vi "UpdateDAQLinescanImage.vi"(2 "Image Settings":refnum<vi>, 3 "buffer (output)":u32[](array[numeric]), 4 "count (read)":u32, 5 "operation":enum16{"initialize", "update", "read"}(ring)) -> (0 "LinescanSampling":T1 {"MacrotimeCycle" format="%.2f"; "OverflowConstant" format="%.2f"; "BinningMicroS" format="%.2f"}, 1 "end of line":bool)   [LabVIEW 2009]
uses:
  ImageSettings.ctt
  ScannedImage.ctl
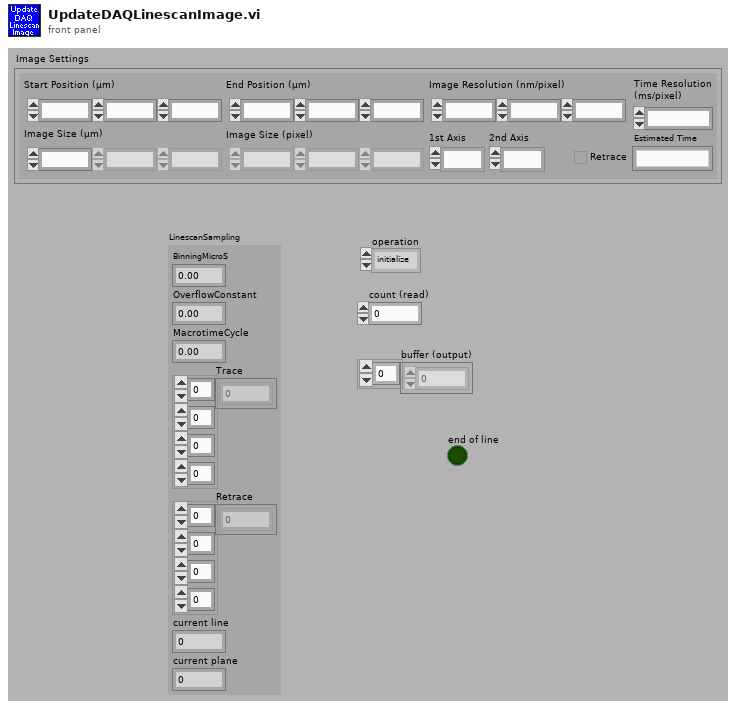
[diagram p1: front panel]
types:
  T1 = typedef "ScannedImage.ctl" = cluster{"BinningMicroS":dbl, "OverflowConstant":dbl, "MacrotimeCycle":dbl, "Trace":u32[][][][], "Retrace":u32[][][][], "current line":i32, "current plane":i32}
  T2 = cluster{"BinningMicroS":dbl, "OverflowConstant":dbl, "MacrotimeCycle":dbl, "Trace":u32[][][][], "Retrace":u32[][][][], "current line":i32, "current plane":i32}
  T3 = typedef "FIFOSettings.ctt" = cluster{"Measurement":cluster{"Binning (ms)":sgl, "External Trigger Condition":u16, "Stop Condition:":u16, "Stop Count":dbl, "Buffer Size (Photons)":u32, "No of Channels":u16, "Ext Latch Delay":i16}, "ADC":cluster{"Binning (HH)":i16, "Dither Range":i16, "Count Increment":i16, "Mode":u16}, "SYNC":cluster{"SYNC ZC Level (mV)":sgl, "SYNC Freq Divider":u16, "SYNC Holdoff (ps)":sgl, "SYNC Threshold (mV)":sgl}, "TAC":cluster{"TAC Range (ns)":sgl, "TAC Gain":i16, "TAC Offset (%)":sgl, "TAC Limit Low (%)":sgl, "TAC Limit High (%)":sgl}, "Ch 2":cluster{"Ch2 ZC Level (mV)":sgl, "Ch2 Holdoff (ps)":sgl, "Ch2 Threshold (mV)":sgl}, "Ch 3":cluster{"Ch3 ZC Level (mV)":sgl, "Ch3 Holdoff (ps)":sgl, "Ch3 Threshold (mV)":sgl}, "Ch 4":cluster{"Ch4 ZC Level (mV)":sgl, "Ch4 Holdoff (ps)":sgl, "Ch4 Threshold (mV)":sgl}, "Ch1":cluster{"Ch1 ZC Level (mV)":sgl, "Ch1 Holdoff (ps)":sgl, "Ch1 Threshold (mV)":sgl}}
  T4 = cluster{"Start Position (µm)":cluster{"x":dbl, "y":dbl, "z":dbl}, "End Position (µm)":cluster{"x":dbl, "y":dbl, "z":dbl}, "Image Resolution (nm/pixel)":cluster{"x":dbl, "y":dbl, "z":dbl}, "Image Size (µm)":cluster{"x":dbl, "y":dbl, "z":dbl}, "Image Size (pixel)":cluster{"x":u32, "y":u32, "z":u32}, "Time Resolution\n(ms/pixel)":dbl, "1st Axis":u16, "2nd Axis":u16, "Retrace":bool, "Estimated Time":string}
  T5 = typedef "LineScanStatus.ctt" = cluster{"in line":bool, "line status":cluster{"count":u32, "current":cluster{"x":u32, "y":u32, "z":u32}}, "plane status":cluster{"count":u32, "current":cluster{"x":u32, "y":u32, "z":u32}}, "new line step":cluster{"x":dbl, "y":dbl, "z":dbl}, "new plane step":cluster{"x":dbl, "y":dbl, "z":dbl}}
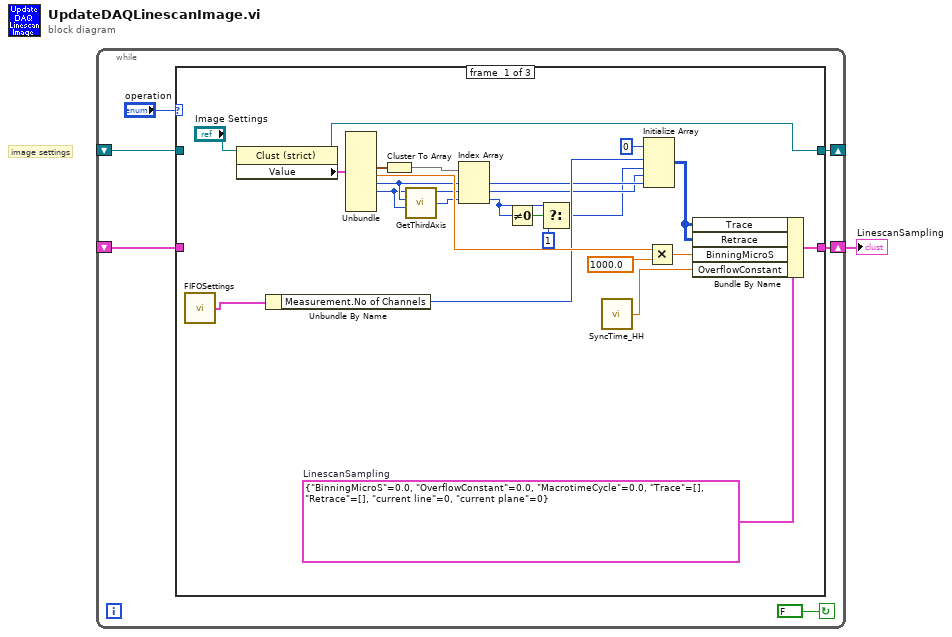
[diagram p0: block diagram]
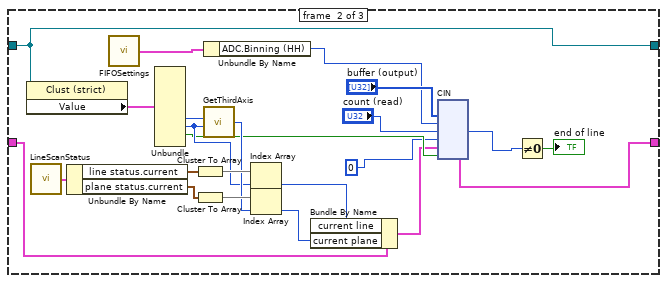
[diagram p2: hidden frame]
diagram:
  # "image settings"
  n1 = while {
    shift-right: [w5] -> w1
    shift-left: _ -> [w4]
    shift-right: [w3] -> _
    shift-left: _ -> [w2]
    stop <- FALSE continue-if-true
    n2 = case shown="\"update\"" "operation" {
      tunnel: [w27 w35 w56] -> w5
      tunnel: w4 -> [_ w43 w56]
      tunnel: [w24 w52 w55] -> w3
      tunnel: w2 -> [_ w52 w55]
      frame #0 {
        w28 = T2 {"BinningMicroS"=0.0, "OverflowConstant"=0.0, "MacrotimeCycle"=0.0, "Trace"=[], "Retrace"=[], "current line"=0, "current plane"=0}  # LinescanSampling
        n3 = call "FIFOSettings.vi"() -> ("FIFO Settings(out)"=w26:T3)  [unwired: 2 in]
        n4 = property class="Clust (strict)"(reference="Image Settings") -> (reference out=w24:refnum<vi>, "Value"=w29:T4)  [unwired: 1 in, 1 out]
        n5 = Unbundle By Name(w26) -> ("Measurement.No of Channels"=w18:u16)
        n6 = Unbundle(w29) -> ("Image Size (pixel)"=w31:cluster{"x":u32, "y":u32, "z":u32}, "Time Resolution\n(ms/pixel)"=w20:dbl, "1st Axis"=w15:u16, "2nd Axis"=w14:u16)  [unwired: 6 out]
        n7 = Cluster To Array(cluster=w31) -> (array=w30:u32[])
        n8 = call "GetThirdAxis.vi"("1st Axis"=w14, "2nd Axis"=w15) -> ("3rd Axis"=w13:i32)  [unwired: 2 in]
        n9 = Index Array(array=w30, index #1=w15, index #2=w14, index #3=w13) -> (element #1=w17:u32, element #2=w16:u32, element #3=w11:u32)
        n10 = Not Equal To 0?(x=w11) -> (x != 0?=w12:bool)
        n11 = Select(t=w11, s=w12, f=u32 1) -> (s? t:f=w9:u32)
        n12 = call "SyncTime_HH.vi"() -> ("OverFlowConstant80Mhz(µs)"=w8:dbl)
        n13 = Initialize Array(u32 0, w18, w9, w16, w17) -> (w22:u32[][][][])
        n14 = Multiply(x=w20, y=1000.0) -> (x*y=w19:dbl)
        n15 = Bundle By Name(cluster=w28, "Trace"=w22, "Retrace"=w22, "BinningMicroS"=w19, "OverflowConstant"=w8) -> (w27:T2)
      }
      frame #1 {
        n16 = property class="Clust (strict)"(reference=w52) -> ("Value"=w53:T4)  [unwired: 1 in, 2 out]
        n17 = call "LineScanStatus.vi"() -> ("Linescan Status (output)"=w50:T5)  [unwired: 2 in]
        n18 = Unbundle By Name(w50) -> ("line status.current"=w48:cluster{"x":u32, "y":u32, "z":u32}, "plane status.current"=w46:cluster{"x":u32, "y":u32, "z":u32})
        n19 = call "FIFOSettings.vi"() -> ("FIFO Settings(out)"=w54:T3)  [unwired: 2 in]
        n20 = Unbundle(w53) -> ("1st Axis"=w51:u16, "2nd Axis"=w44:u16, "Retrace"=w37:bool)  [unwired: 7 out]
        n21 = Cluster To Array(cluster=w48) -> (array=w49:u32[])
        n22 = Cluster To Array(cluster=w46) -> (array=w47:u32[])
        n23 = Unbundle By Name(w54) -> ("ADC.Binning (HH)"=w39:i16)
        n24 = call "GetThirdAxis.vi"("1st Axis"=w44, "2nd Axis"=w51) -> ("3rd Axis"=w45:i32)  [unwired: 2 in]
        n25 = Index Array(array=w49, index=w44) -> (element=w42:u32)
        n26 = Index Array(array=w47, index=w45) -> (element=w41:u32)
        n27 = Bundle By Name(cluster=w43, "current line"=w42, "current plane"=w41) -> (w36:T2)
        n28 = cin("buffer (output)", w39, "count (read)", u32 0, w36, w37) -> (w33:u32, w35:T2)  [unwired: 4 in]
        n29 = Not Equal To 0?(x=w33) -> (x != 0?=→"end of line":bool)
      }
      frame #2 {
      }
    }
  }
  "LinescanSampling" <- w1
